vi "Renishaw-XL80_Init.vi"(8 "error in (no error)":errorcluster, 11 "Renishaw-XL80 in":refnum<class "Renishaw-XL80.lvclass">) -> (0 "error out":errorcluster, 1 "Serial Number":string, 2 "Connect":bool, 3 "Renishaw-XL80 out":refnum<class "Renishaw-XL80.lvclass">)   [LabVIEW 2024, in "Renishaw-XL80.lvclass"]
doc: "This method connects a client to a laser measurement system.\n\nDefinition\nHRESULTConnect( [in, out] BSTR* pbstrSerNum, [out, retval] VARIANT_BOOL* pOk);\nParameters\npbstrSerNum\nDepending on your application this parameter can be used in several ways. On entry it can be set to the serial number of a specific XL laser or DX10 device to connect. It can also be blank, in which case we connect to the first available XL laser, if no laser is available we connect to the first available DX10, finally if there is no DX10 present we will connect to the first available XC weatherstation. Alternatively this can be used as a connection string to associate a specific XL laser with a specific XC compensator device, using the format \"XL:xxxxxx,XC:xxxxxx\" where xxxxxx are the serial number of each device. On return this is set to either the serial number of the DX10 which is connected, or the qualified string for the connected laser system e.g. \"XL:xxxxxx,XC:xxxxxx \"\n\npOk\nA variable that will be set to VARIANT_TRUE or VARIANT_FALSE. If the variable is set to VARIANT_TRUE then the client has successfully connected to either a XL laser or DX10 device.\n\nComments\nThis method should be called before any other property or method. Most of the other methods supported by this interface will return E_FAIL if the client has not already connected. The client should keep trying to connect until it succeeds.\n\nThe method will usually return a HRESULT of S_OK. However, it will return E_POINTER if the client supplies null pointers for either pOk or pbstrSerNum, and in extremely low memory conditions it will return E_NOMEMORY.\n\nThe method may fail to connect a client to a laser system under any of the following conditions:\n\nthe client specified a XL laser system or DX10 that is not attached to the PC \nthere are no XL lasers, DX10s, or XC weatherstations attached to the PC \nall XL laser systems and DX10s attached to the PC are connected to other clients. \nNote that if the client has already connected to either a XL laser or DX10 then this method will succeed. It will set pOk to VARIANT_TRUE and set pbstrSerNum to the serial number or qualified string of the connected devices.\n\nIf this method successfully connects to a XL laser we return a pOk of VARIANT_TRUE regardless of the XC compensator's connection status. We will continue to poll the XC for connection and return a status of EC10_NOT_RESPONDING. If the XC's serial number is not specified as in the connection string above, any available XC will be connected and associated with the XL laser.\n\nIf this method successfully connects to a XC weatherstation we return a pOk of VARIANT_TRUE regardless of the XL laser's connection status. We will continue to poll the XL for connection and return a status of ML10_NOT_RESPONDING. If the XL's serial number is not specified as in the connection string above, any available XL will be connected and associated with the XC weatherstation. \n\nIt is important that the client application calls Disconnect before it exits. For most languages this will be done automatically when the last reference to the COM object is released, but we have found some, notably C#, that wait until garbage collection to release the COM object. Garbage collection may occur at any time. This can mean that the DX10 remains unavailable to other clients.\n\nA similar effect may occur if the client crashes before calling Disconnect. In both cases, if you are connected to a DX10, restarting DX10Server.exe is the only way to recover."
uses:
  Renishaw-XL80.lvclass
  Renishaw-XL80.lvclass/Renishaw-XL80.ctl
  D:/A.C.M/Example CSharp_64/bin/Debug/Interop.DX10SDKADAPTORLib.dll
  Example CSharp_64/bin/Debug/Interop.DX10SDKADAPTORLib.dll
panel:
  out "IsConnected":bool
  out "DX10SerialNumber":string
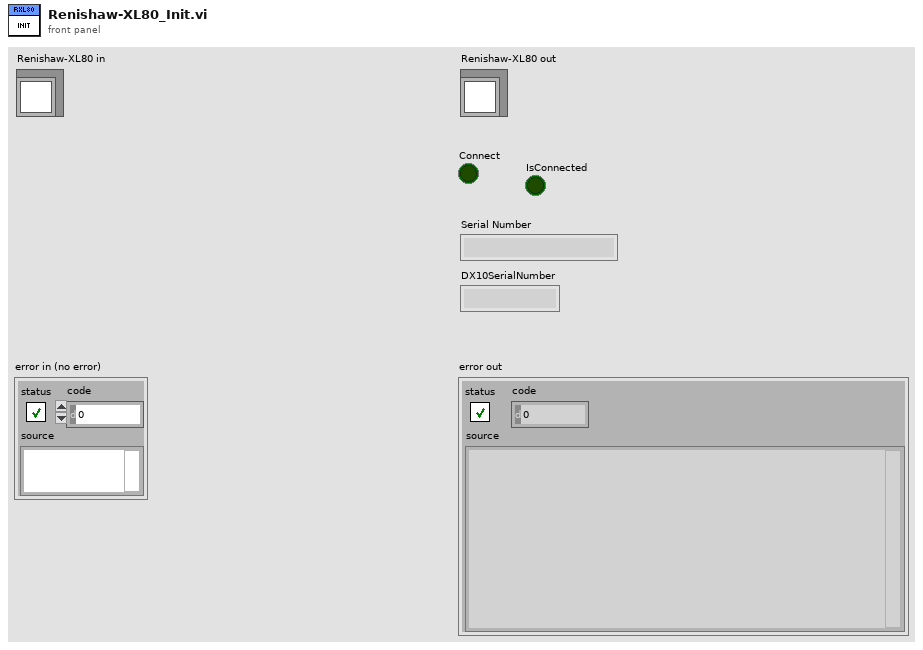
[diagram p1: front panel]
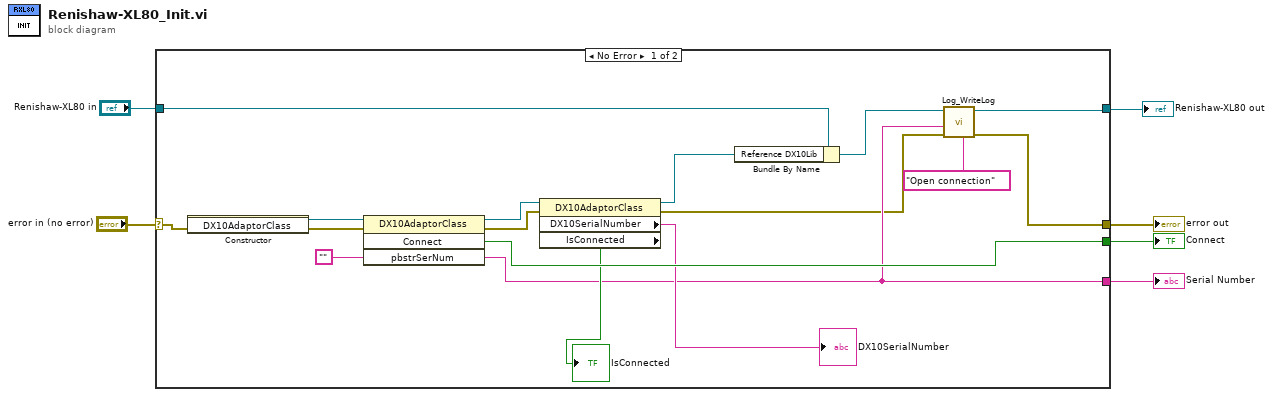
[diagram p0: block diagram]
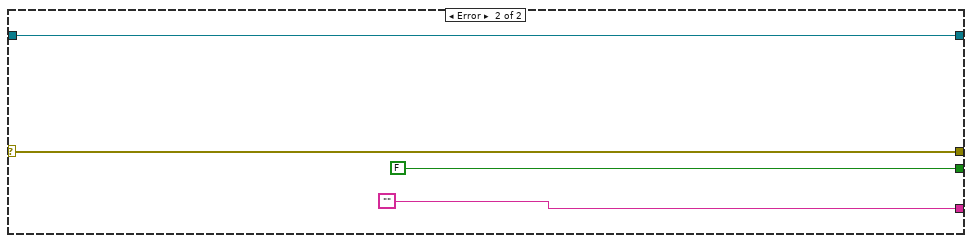
[diagram p2: hidden frame]
diagram:
  n1 = case shown="No Error" "error in (no error)" {
    selector: "error in (no error)" -> [w18 w27]
    tunnel: [w11 w27] -> w5
    tunnel: [w12 w26] -> w3
    tunnel: "Renishaw-XL80 in" -> [w19 w26]
    tunnel: [w9 ""] -> w2
    tunnel: [w20 FALSE ("Connect")] -> w1
    frame No Error {
      n2 = constructor class="DX10AdaptorClass"(error in=w18) -> (reference out=w22:refnum<k24>, error out=w23:errorcluster)  [unwired: 2 in, 1 out]
      n3 = invoke class="DX10AdaptorClass" method="Connect"(reference=w22, error in=w23, "pbstrSerNum"="") -> (reference out=w17:refnum<k24>, error out=w8:errorcluster, "Connect"=w20:bool, "pbstrSerNum"=w9:string)  [unwired: 1 in]
      n4 = property class="DX10AdaptorClass"(reference=w17, error in=w8) -> (reference out=w16:refnum<k24>, error out=w7:errorcluster, "DX10SerialNumber"=→"DX10SerialNumber":string, "IsConnected"=→"IsConnected":bool)
      n5 = Bundle By Name(cluster=w19, "Reference DX10Lib"=w16) -> (w13:refnum<class "Renishaw-XL80.lvclass">)
      n6 = call-dynamic "Log_WriteLog.vi"("Additional text"="Open connection", "error in (no error)"=w7, "Response"=w9, "Log in"=w13) -> ("error out"=w11:errorcluster, "Log out"=w12:refnum<class "Renishaw-XL80.lvclass">)  [unwired: 6 in]
    }
    frame Error {
    }
  }
  "error out" <- w5
  "Renishaw-XL80 out" <- w3
  "Connect" <- w1
  "Serial Number" <- w2
